vi "Omega read sensor.vi"() -> (0 "Stop":bool, 1 "Current Reading":dbl[](array[numeric]))   [LabVIEW 2019]
doc: "This VI returns the value of CNi32 Current Reading from the Omega Temp Server VI in a format compatable with NHMFL Data Acquisition. Adapted from code by Scott Hannahs.\nJonathan Billings, NHMFL-FSU, Jan 2008"
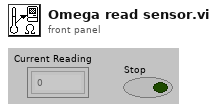
[diagram p1: front panel]
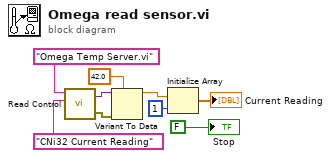
[diagram p0: block diagram]
diagram:
  n1 = call "Read Control.vi"("VI Name"="Omega Temp Server.vi", "Control Name"="CNi32 Current Reading") -> ("Value"=w5:variant, "error out"=w4:errorcluster)  [unwired: 3 in]
  n2 = Variant To Data(error in=w4, type=42.0, Variant=w5) -> (data=w9:dbl)  [unwired: 1 out]
  n3 = Initialize Array(w9, 1 ("dimension size")) -> (→"Current Reading":dbl[])
  "Stop" <- FALSE
